vi "Primative_Duty_Cycle.vi"(3 "Input power":dbl) -> (0 "Duty cycle acheived":dbl, 1 "Mins on":i32[](array[numeric]))   [LabVIEW 2011]
panel:
  out "size(s)":i32
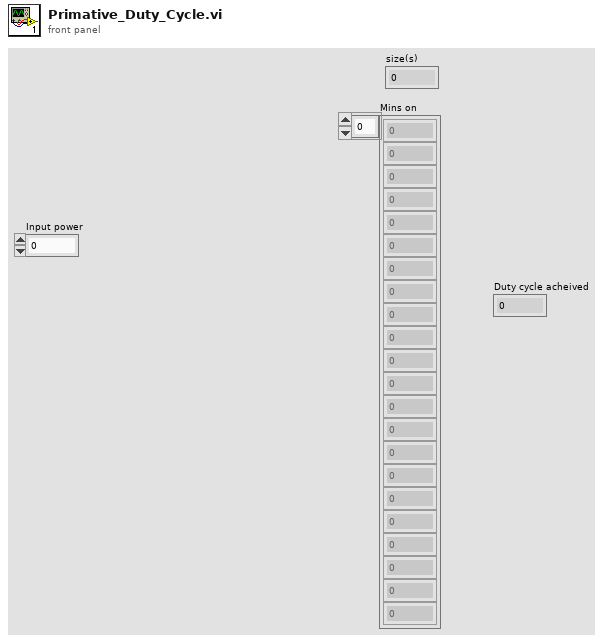
[diagram p1: front panel]
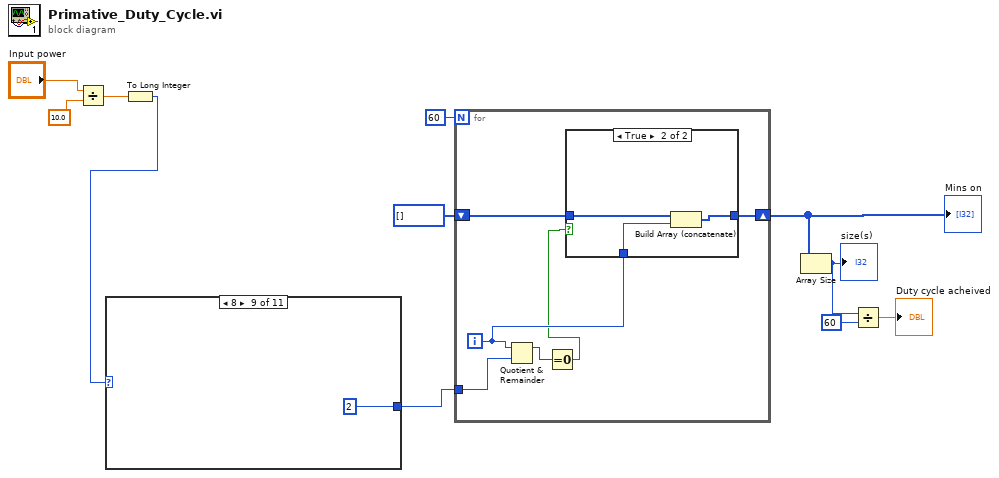
[diagram p0: block diagram]
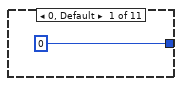
[diagram p2: hidden frame]
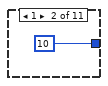
[diagram p3: hidden frame]
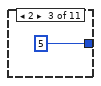
[diagram p4: hidden frame]
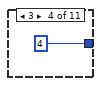
[diagram p5: hidden frame]
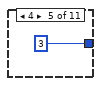
[diagram p6: hidden frame]
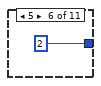
[diagram p7: hidden frame]
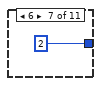
[diagram p8: hidden frame]
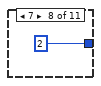
[diagram p9: hidden frame]
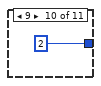
[diagram p10: hidden frame]
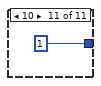
[diagram p11: hidden frame]
diagram:
  n1 = Divide(x="Input power", y=10.0) -> (x/y=w3:dbl)
  n2 = To Long Integer(number=w3) -> (32bit integer=w2:i32)
  n3 = case shown="8" w2 {
    tunnel: [0 10 5 4 3 2 2 2 2 2 1] -> w1
    frame 0, Default {
    }
    frame 1 {
    }
    frame 2 {
    }
    frame 3 {
    }
    frame 4 {
    }
    frame 5 {
    }
    frame 6 {
    }
    frame 7 {
    }
    frame 8 {
    }
    frame 9 {
    }
    frame 10 {
    }
  }
  n4 = for {
    N: 60 -> [_]
    shift-right: [w26] -> w7
    shift-left: i32[] [] -> [w27]
    tunnel: w1 -> [w25]
    i -> [w28]
    n5 = Quotient & Remainder(x=w28, y=w25) -> (x-y*floor(x/y)=w24:i32)  [unwired: 1 out]
    n6 = Equal To 0?(x=w24) -> (x = 0?=w23:bool)
    n7 = case shown="True" w23 {
      tunnel: w28 -> [_ w30]
      tunnel: w27 -> [w29 w32]
      tunnel: [w29 w31] -> w26
      frame False {
      }
      frame True {
        n8 = Build Array (concatenate)(w32, w30) -> (w31:i32[])
      }
    }
  }
  "Mins on" <- w7
  n9 = Array Size(array=w7) -> (size(s)=w6:i32)
  "size(s)" <- w6
  n10 = Divide(x=w6, y=60) -> (x/y=→"Duty cycle acheived":dbl)
